vi "ExtractReply.vi"(8 "error in (no error)":errorcluster, 11 "Message Data in":variant) -> (0 "error out":errorcluster, 2 "Reply Payload":T1, 3 "Message Data out":variant)   [LabVIEW 2024, in "ModuleQueue.lvclass"]
uses:
  ModuleQueue.lvclass
  ModuleCore/Reply.ctl
  ModuleCore/Module.lvclass
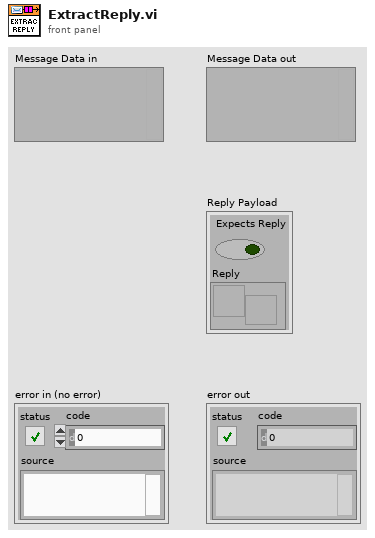
[diagram p1: front panel]
types:
  T1 = typedef "Module.lvclass/Reply.ctl" = cluster{"Expects Reply":bool, "Reply":refnum<notifier>}
  T2 = cluster{"Message Data":variant, "Reply Payload":T1}
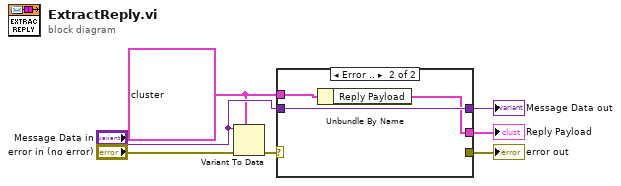
[diagram p0: block diagram]
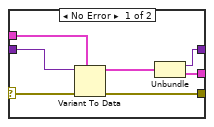
[diagram p2: hidden frame]
diagram:
  w2 = T2 {"Message Data"=variant, "Reply Payload"={"Expects Reply"=FALSE, "Reply"=refnum}} ("cluster")
  n1 = Variant To Data(error in="error in (no error)", type=w2, Variant="Message Data in") -> (error out=w1:errorcluster)  [unwired: 1 out]
  n2 = case shown="Error .." w1 {
    selector: w1 -> [w14 _]
    tunnel: w2 -> [w13 w16]
    tunnel: "Message Data in" -> [w12 w17]
    tunnel: [w11 _] -> w4
    tunnel: [w9 w17] -> w5
    tunnel: [w8 w15] -> w6
    frame No Error {
      n3 = Variant To Data(error in=w14, type=w13, Variant=w12) -> (data=w10:T2, error out=w11:errorcluster)
      n4 = Unbundle(w10) -> ("Message Data"=w9:variant, "Reply Payload"=w8:T1)
    }
    frame Error {
      n5 = Unbundle By Name(w16) -> ("Reply Payload"=w15:T1)
    }
  }
  "Reply Payload" <- w6
  "Message Data out" <- w5
  "error out" <- w4
